vi "DropletDB-GFV.vi"(8 "error in (no error)":errorcluster, 9 "Droplets Proccesed":refnum<vi>, 10 "Data in":variant, 11 "Command In":T2=enum."Init") -> (0 "error out":errorcluster, 2 "Data out":variant)   [LabVIEW 2013]
uses:
  DbEnum.ctl
  TypeDef/MatchesAndCircles.ctl
  ConfEnum.ctl
  ConfDB.ctl
  TypeDef/Magnification.ctl
  TypeDef/GreyLevelData.ctl
  TypeDef/FreezePointData.ctl
  DropletDB.ctl
panel:
  out "Image Out 3":T1(plugin-control)
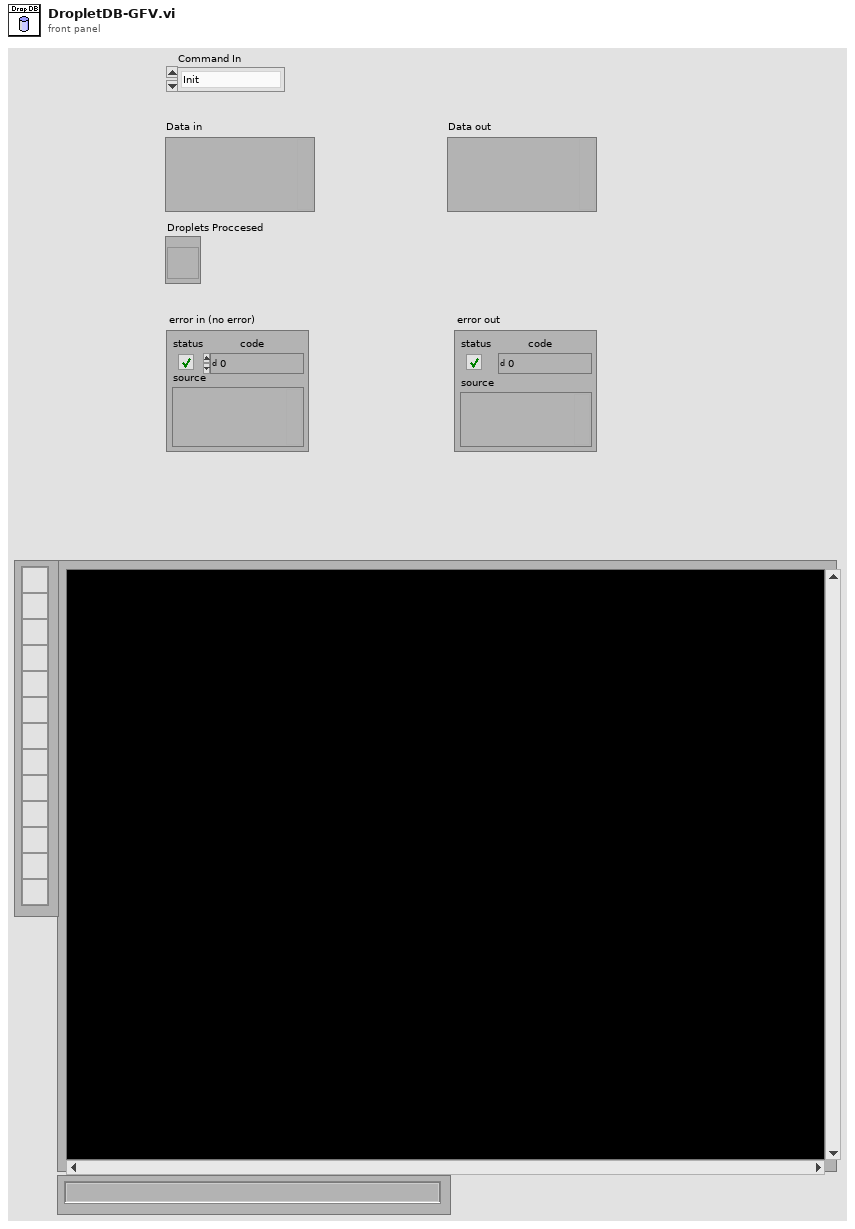
[diagram p1: front panel]
types:
  T1 = typedef "IMAQ Image.ctl" = refnum<image>
  T2 = typedef "DbEnum.ctl" = enum16{"RemoveOneDroplet", "AddOneDroplet", "Write DropletDB", "Init", "Insert Detection Result Data", "Insert Grey Level Result", "Insert Baseline Results", "AddFreezeImagesAtCertainDroplet", "UpdateIncludeDroplet", "Insert Freeze Analysis Results", "GetDropDB", "GetNoFreezedDroplets", "GetGreyLevelAndDiff", "GetGreyLevelatIndexTime", "GetDropletsBoundingBox", "GetDropletsDiameter"}
  T3 = typedef "ConfDB.ctl" = cluster{"NumberOfImages":i32, "NoImages2SaveAroundFreeze":i32, "Path":path, "NameOfPartialFile":string, "StartIndex":i32, "NumberOfStdTol":i32, "Detla t (sec)":i32, "Number of images for baseline":i32, "Temperature File Name":string, "Score":dbl, "Index number of Files":i32[], "End Index":i32, "Temperature Array":dbl[], "TStartIndex":i32, "Magnification (Microns/Pixel)":T4, "Circle Descriptor":cluster{"Min Radius":dbl, "Max Radius":dbl}}
  T4 = typedef "Magnification.ctl" = dbl
  T5 = typedef "ConfEnum.ctl" = enum16{"Init", "GetConfDB", "GetTemperatureAtIndex", "WriteConfDB", "Configure DB"}
  T6 = typedef "DropletDB.ctl" = cluster{"ImageFreezeIndex":i32, "DropIndex":i32, "Position":cluster{"x":sgl, "y":sgl}, "Bounding Box":cluster{"x":sgl, "y":sgl}[], "Score":sgl, "GreyLevelInBoundingBox":dbl[], "GLDifference":dbl[], "Baseline level":dbl, "Peak":cluster{"Value":dbl, "Index":u32}, "Peak Onset":cluster{"Value":dbl, "Index":u32}, "FreezeFileName":string, "FreezeAbsTime":timestamp, "FreezeTemperature":dbl, "ImageIndexArray":u32[], "Freeze Point Found":bool, "Baseline std":dbl, "FreezedImageArray":cluster{"Image":u8[][]}[], "Include Droplet":bool, "Remark":string, "Freeze Rel Time":u32[], "Diameter (microns)":dbl}[]
  T7 = typedef "GreyLevelData.ctl" = cluster{"Grey Level":dbl[], "Grey level diff":dbl[], "ImageIndex":u32, "Drop Index":u32}
  T8 = typedef "FreezePointData.ctl" = cluster{"Freeze YesNo":cluster{"Freeze Grey Diff value":dbl, "Freeze Point Found":bool, "Freeze Indices":u32[]}[], "Rel Time":u32[]}
  T9 = cluster{"DropletBaseline":dbl[], "DropletBaselineSTD":dbl[]}
  T10 = typedef "MatchesAndCircles.ctl" = cluster{"Matches (pixel)":cluster{"Position":cluster{"x":sgl, "y":sgl}, "Angle":sgl, "Scale":sgl, "Score":sgl, "Bounding Box":cluster{"x":sgl, "y":sgl}[]}[], "Circles (Calibrated)":cluster{"Position":cluster{"X":sgl, "Y":sgl}, "Radius":dbl, "Score":dbl}[]}
  T11 = cluster{"Position":cluster{"x":sgl, "y":sgl}, "Angle":sgl, "Scale":sgl, "Score":sgl, "Bounding Box":cluster{"x":sgl, "y":sgl}[]}[]
  T12 = cluster{"Position":cluster{"X":sgl, "Y":sgl}, "Radius":dbl, "Score":dbl}[]
  T13 = cluster{"ImageFreezeIndex":i32, "DropIndex":i32, "Position":cluster{"x":sgl, "y":sgl}, "Bounding Box":cluster{"x":sgl, "y":sgl}[], "Score":sgl, "GreyLevelInBoundingBox":dbl[], "GLDifference":dbl[], "Baseline level":dbl, "Peak":cluster{"Value":dbl, "Index":u32}, "Peak Onset":cluster{"Value":dbl, "Index":u32}, "FreezeFileName":string, "FreezeAbsTime":timestamp, "FreezeTemperature":dbl, "ImageIndexArray":u32[], "Freeze Point Found":bool, "Baseline std":dbl, "FreezedImageArray":cluster{"Image":u8[][]}[], "Include Droplet":bool, "Remark":string, "Freeze Rel Time":u32[], "Diameter (microns)":dbl}
  T14 = cluster{"Global Rectangle":i32[], "Contours":cluster{"Contour Type":u32, "ROI Type":u32, "Points":i32[]}[]}
  T15 = typedef "IMAQ Circle" = cluster{"Center X":i32, "Center Y":i32, "Inner Radius":i32, "Outer Radius":i32, "Start Angle":dbl, "End Angle":dbl}
  T16 = cluster{"Freeze Grey Diff value":dbl, "Freeze Point Found":bool, "Freeze Indices":u32[]}[]
  T17 = cluster{"ImageFreezeIndex":i32, "DropIndex":i32, "Position":cluster{"x":sgl, "y":sgl}, "Bounding Box":cluster{"x":sgl, "y":sgl}[], "Score":sgl, "GreyLevelInBoundingBox":dbl[], "GLDifference":dbl[], "Baseline level":dbl, "Peak":cluster{"Value":dbl, "Index":u32}, "Peak Onset":cluster{"Value":dbl, "Index":u32}, "FreezeFileName":string, "FreezeAbsTime":timestamp, "FreezeTemperature":dbl, "ImageIndexArray":u32[], "Freeze Point Found":bool, "Baseline std":dbl, "FreezedImageArray":cluster{"Image":u8[][]}[], "Include Droplet":bool, "Remark":string, "Freeze Rel Time":u32[], "Diameter (microns)":dbl}[]
  T18 = cluster{"ImageIndexArray":u32[], "GreyLevelInBoundingBox":dbl[][], "GLDifference":dbl[][]}
  T19 = typedef "Image Type" = u32
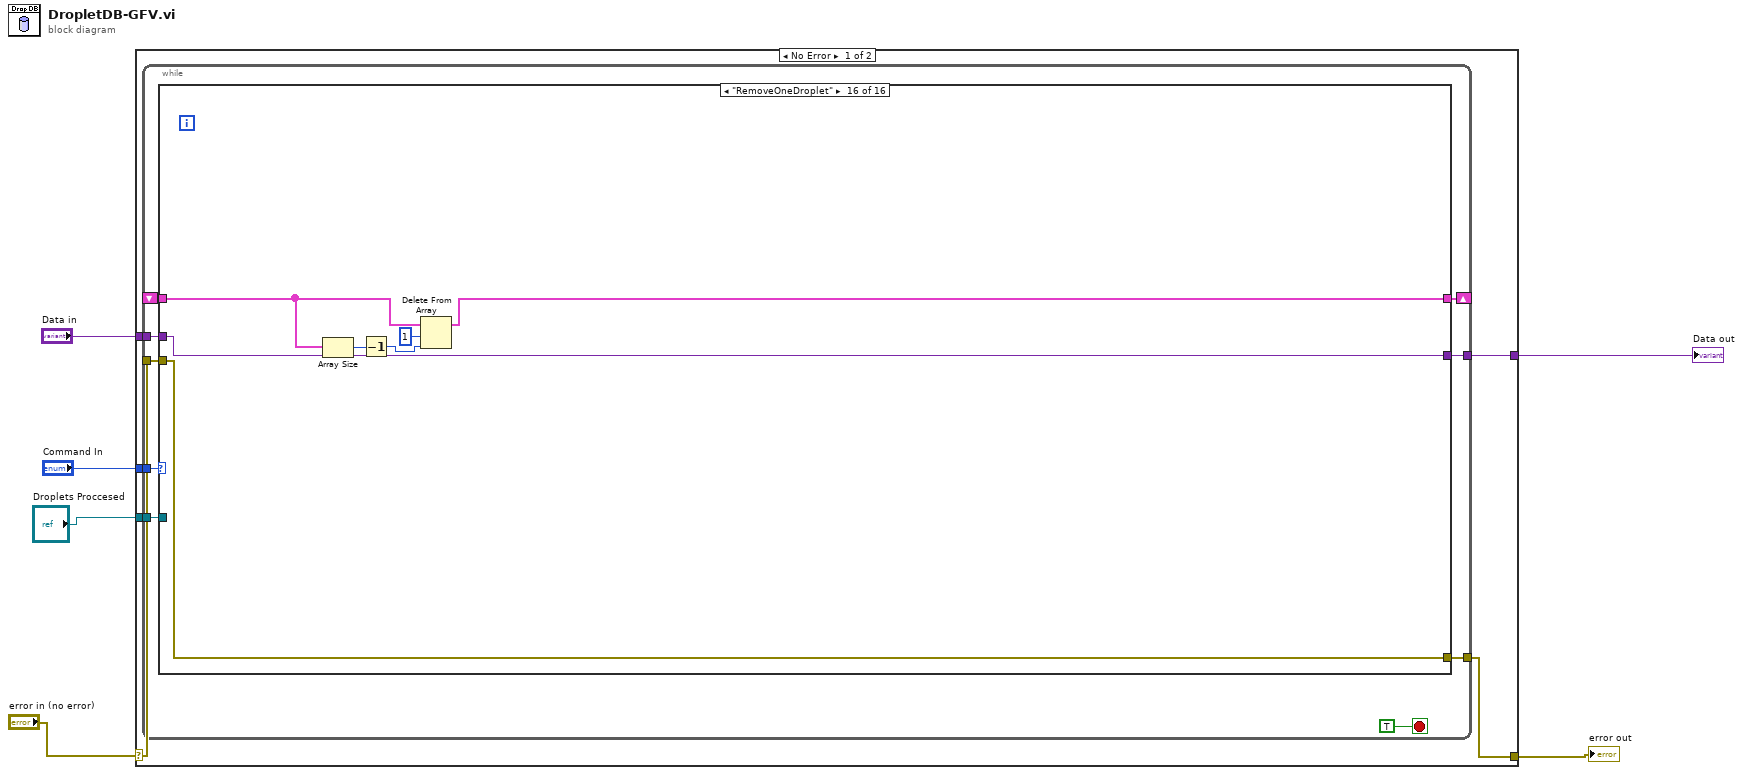
[diagram p0: block diagram]
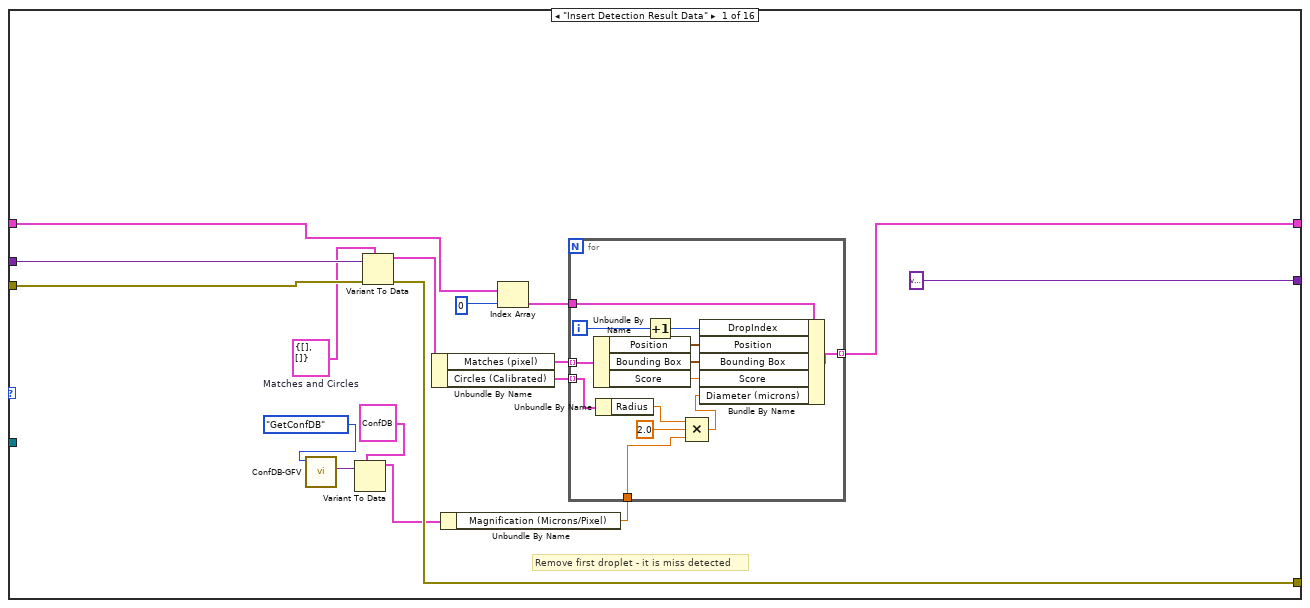
[diagram p2: hidden frame]
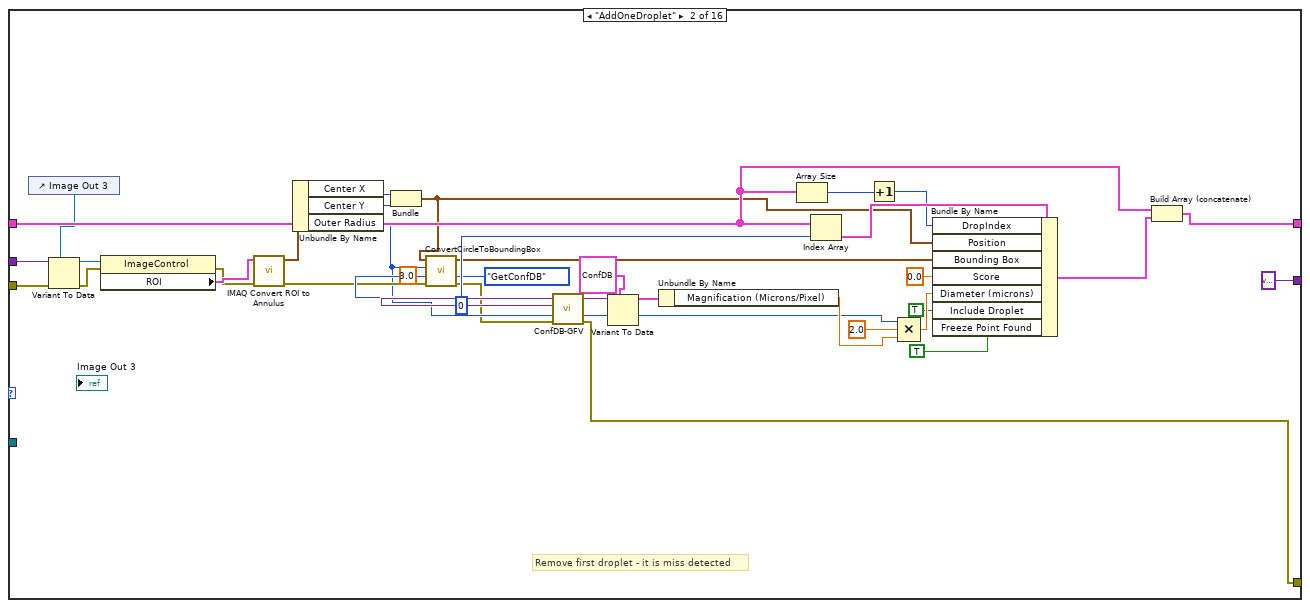
[diagram p3: hidden frame]
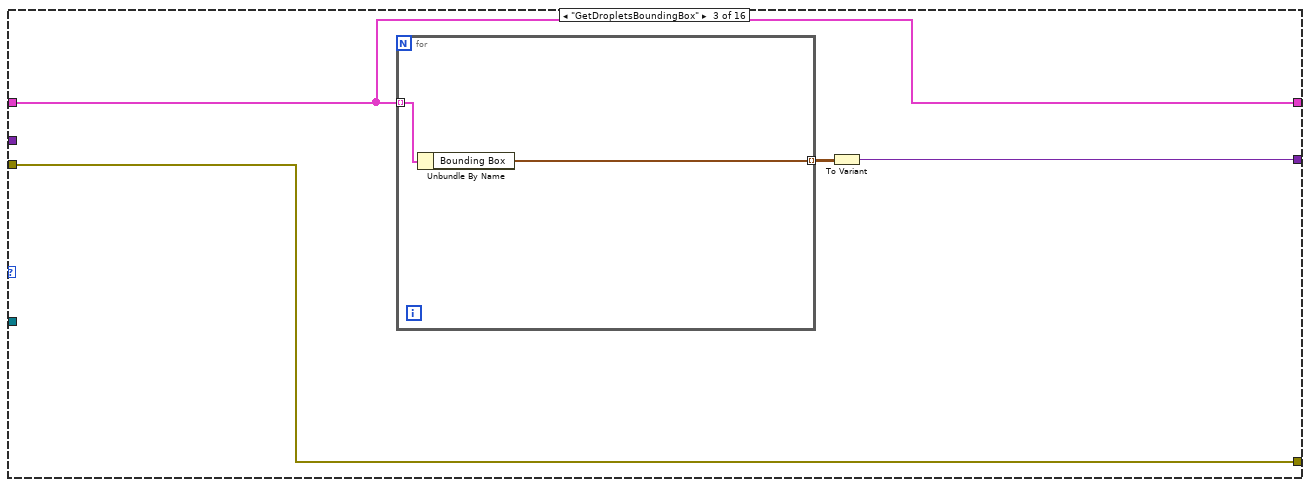
[diagram p4: hidden frame]
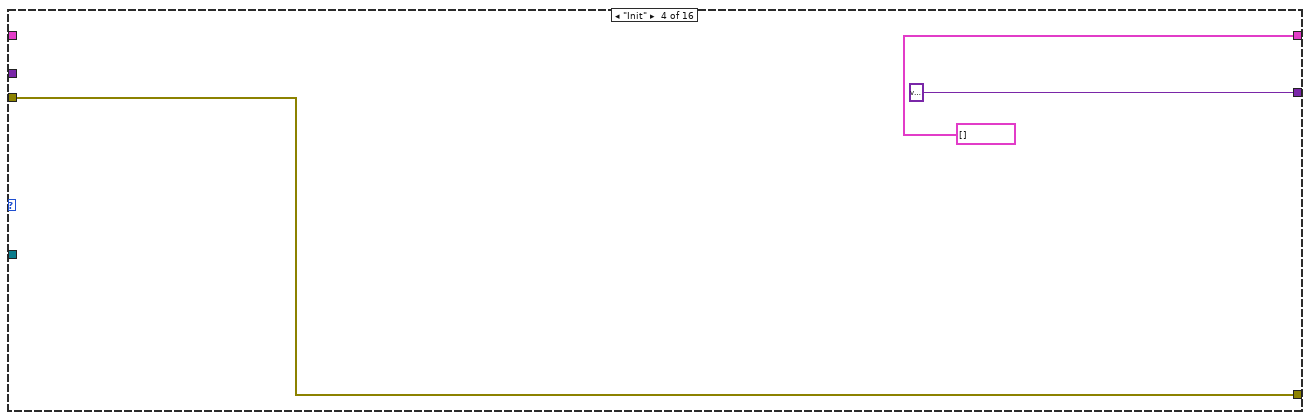
[diagram p5: hidden frame]
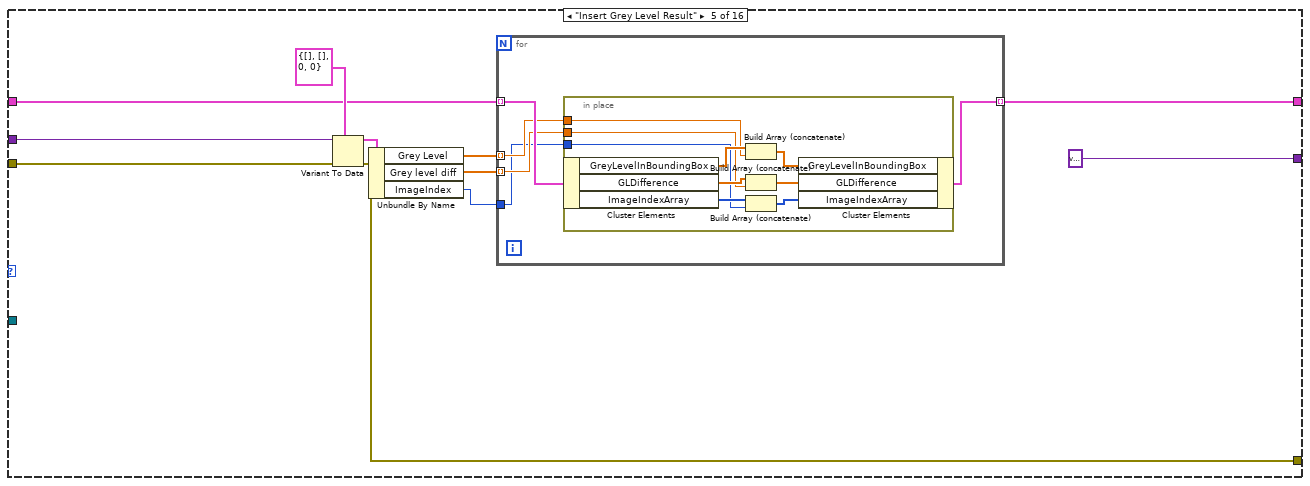
[diagram p6: hidden frame]
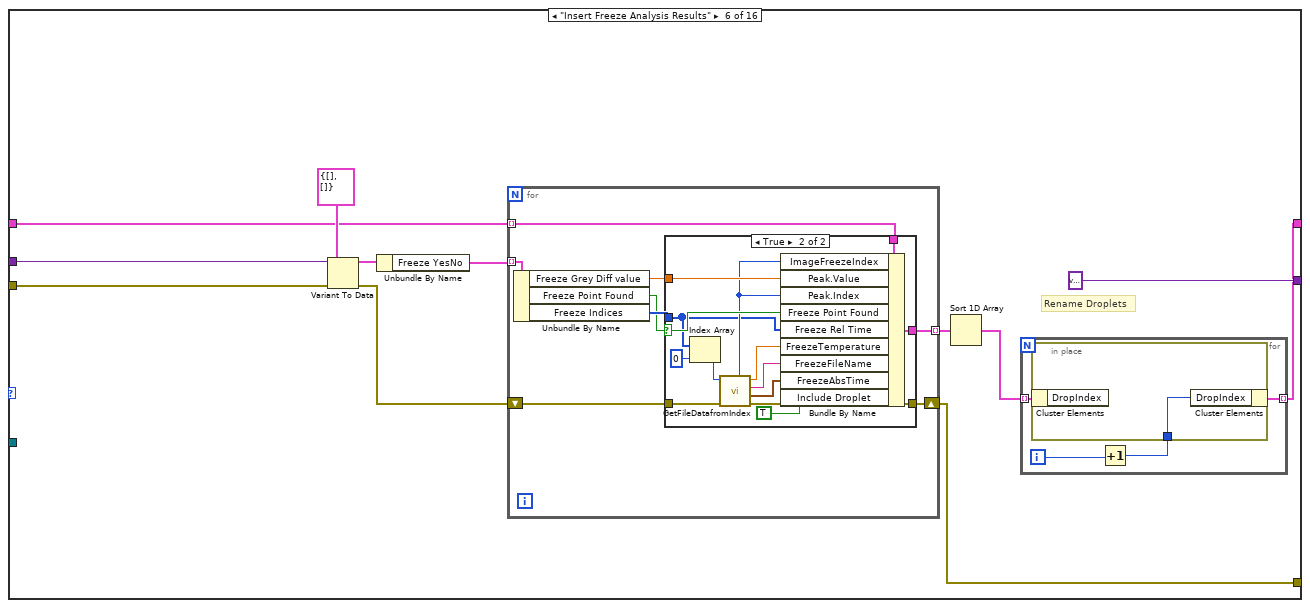
[diagram p7: hidden frame]
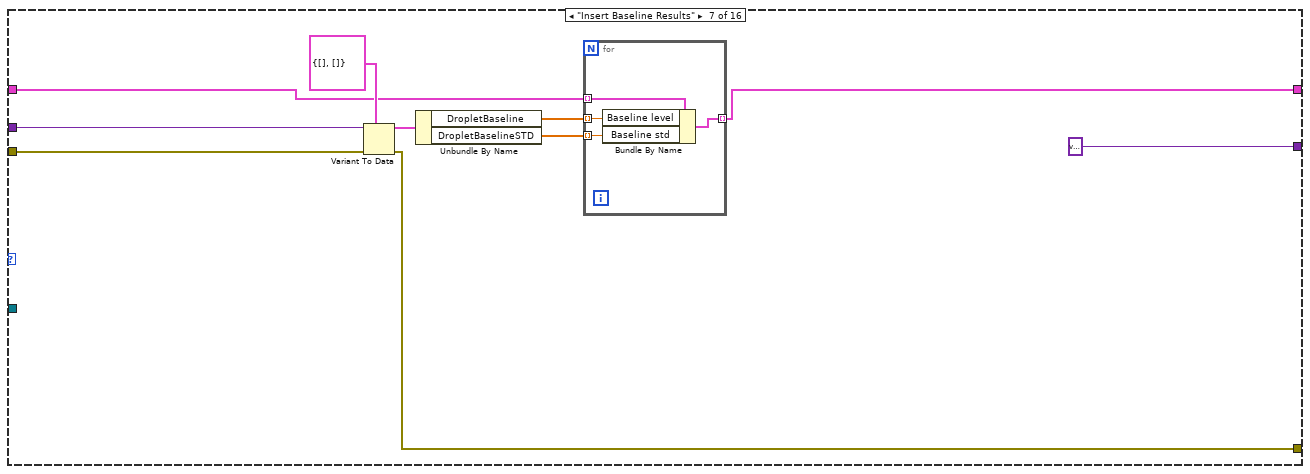
[diagram p9: hidden frame]
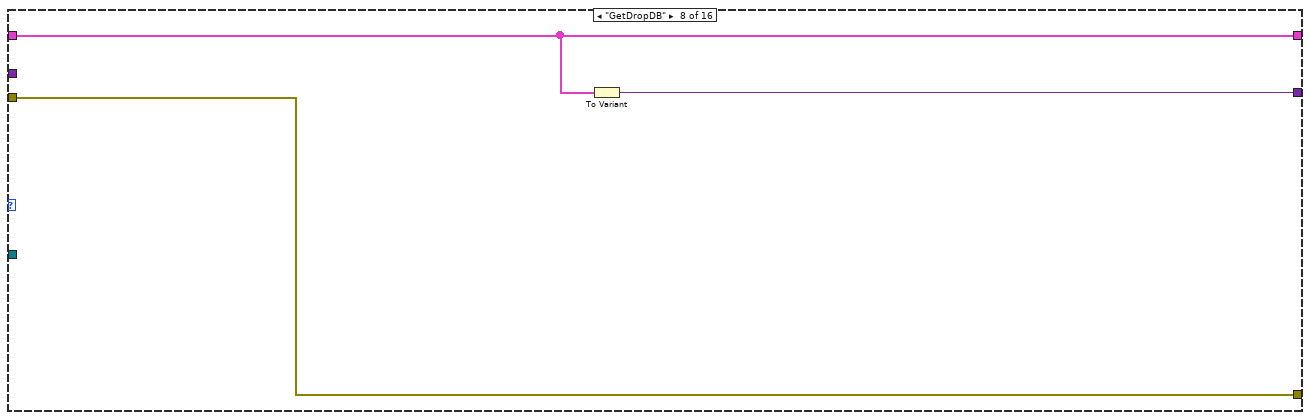
[diagram p10: hidden frame]
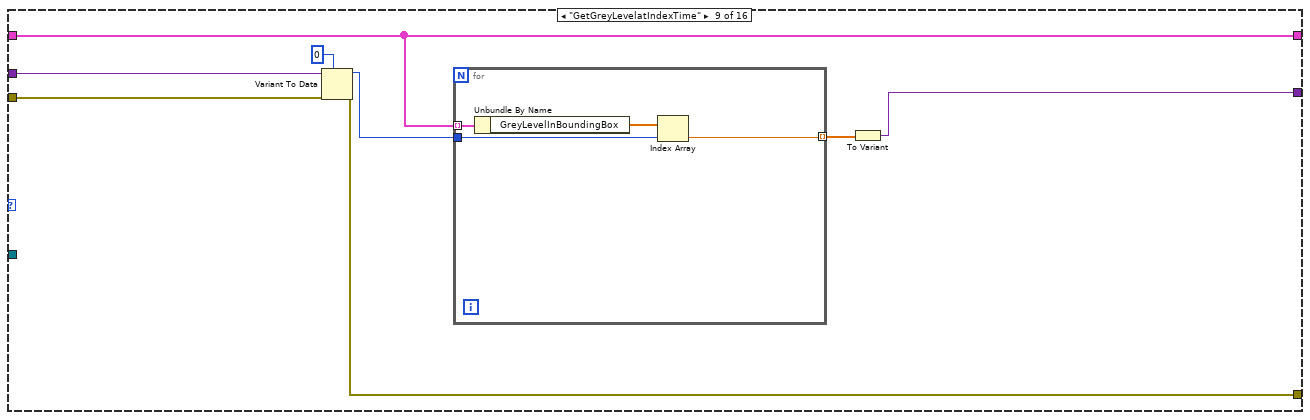
[diagram p11: hidden frame]
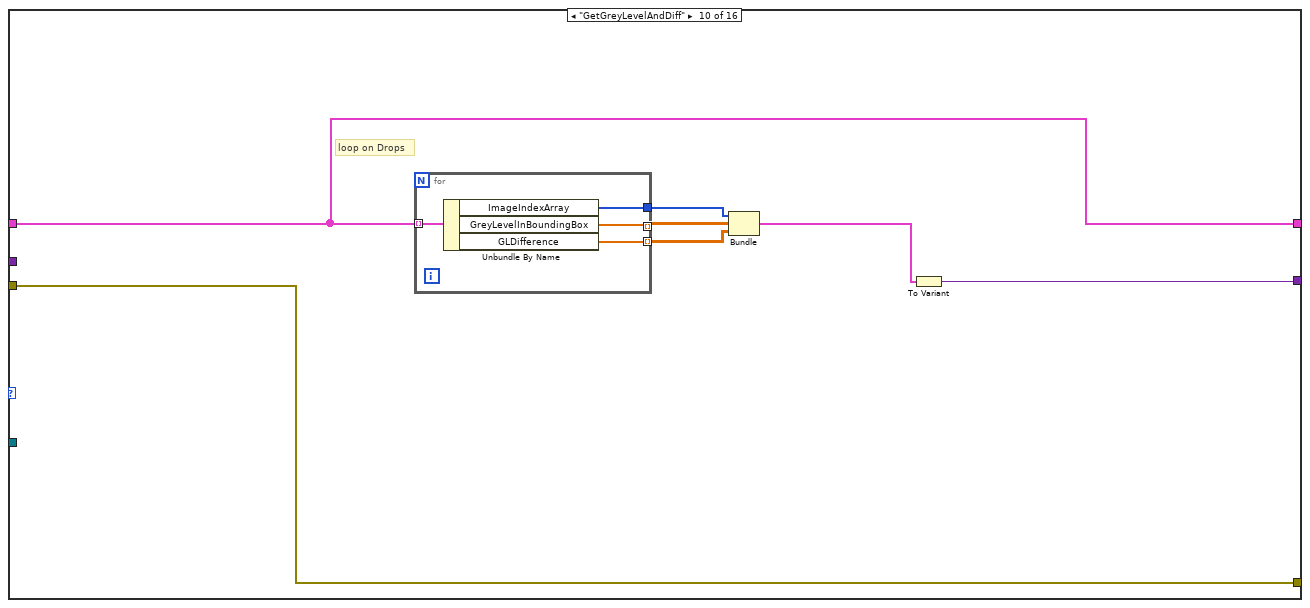
[diagram p12: hidden frame]
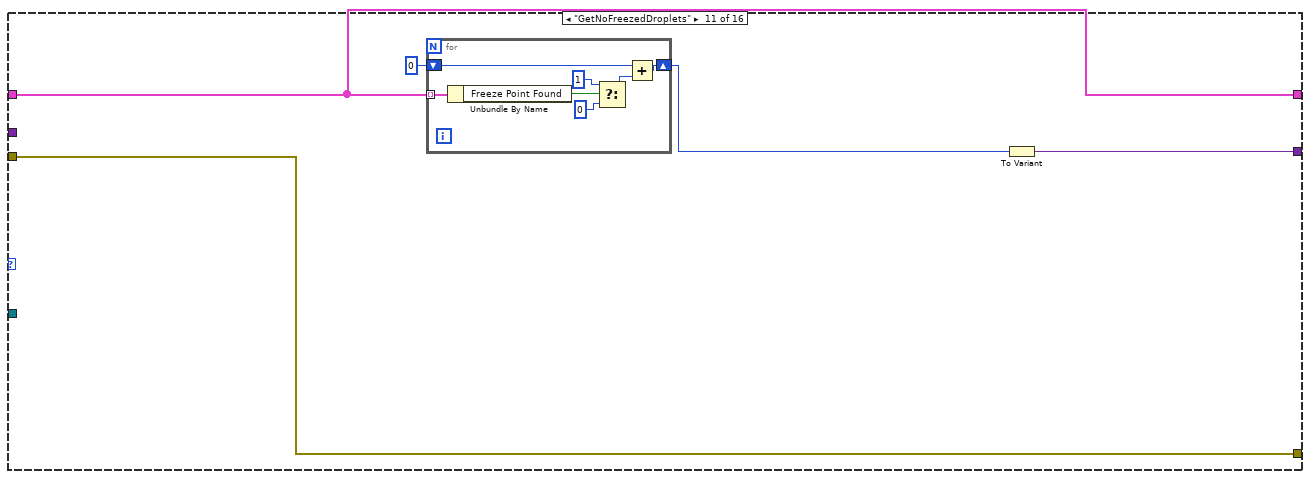
[diagram p13: hidden frame]
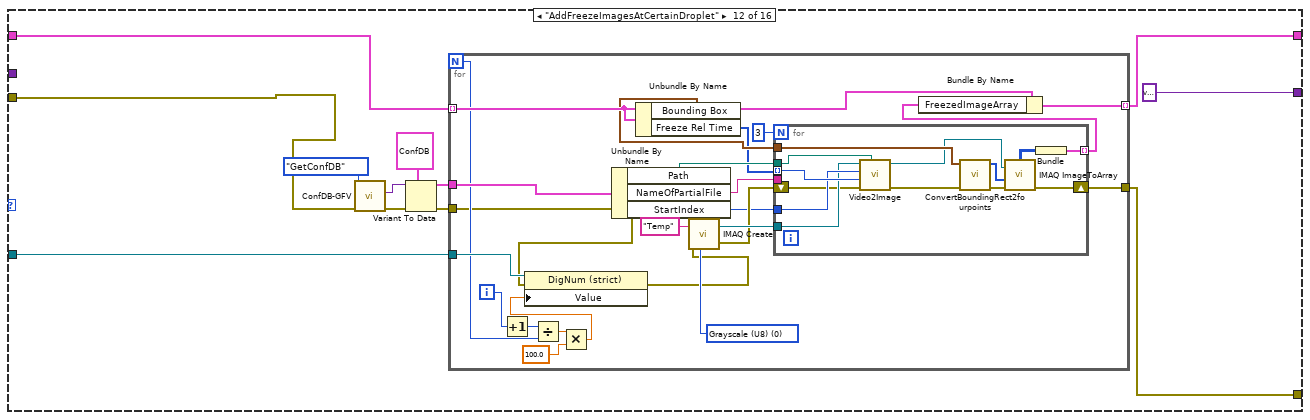
[diagram p14: hidden frame]
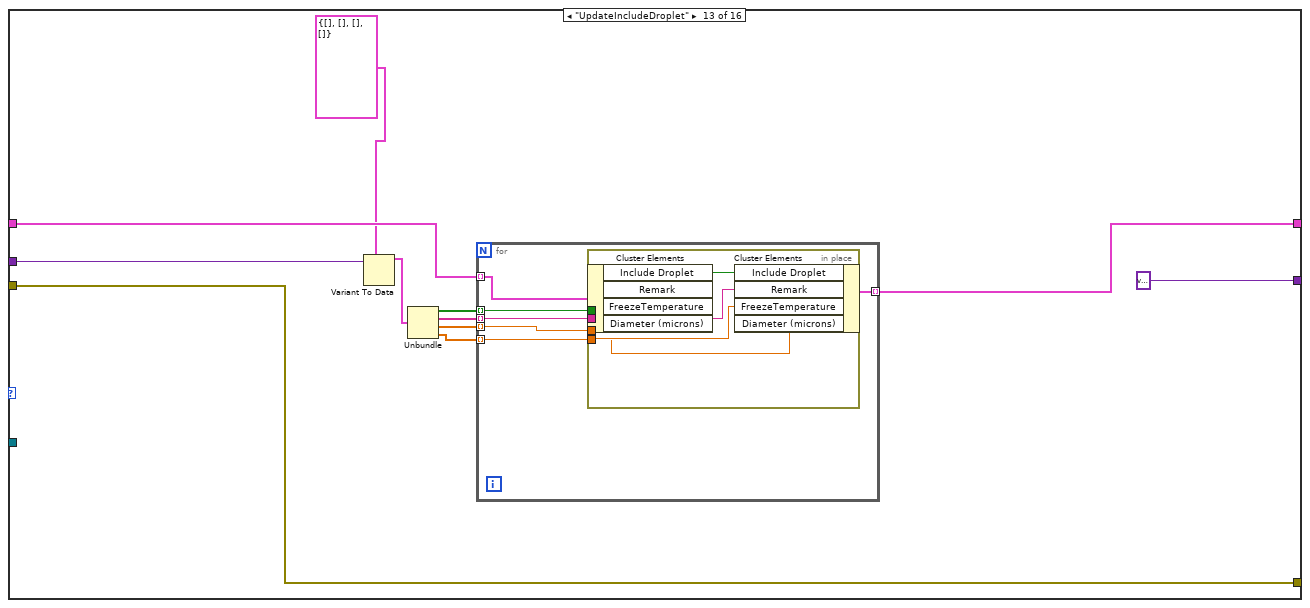
[diagram p15: hidden frame]
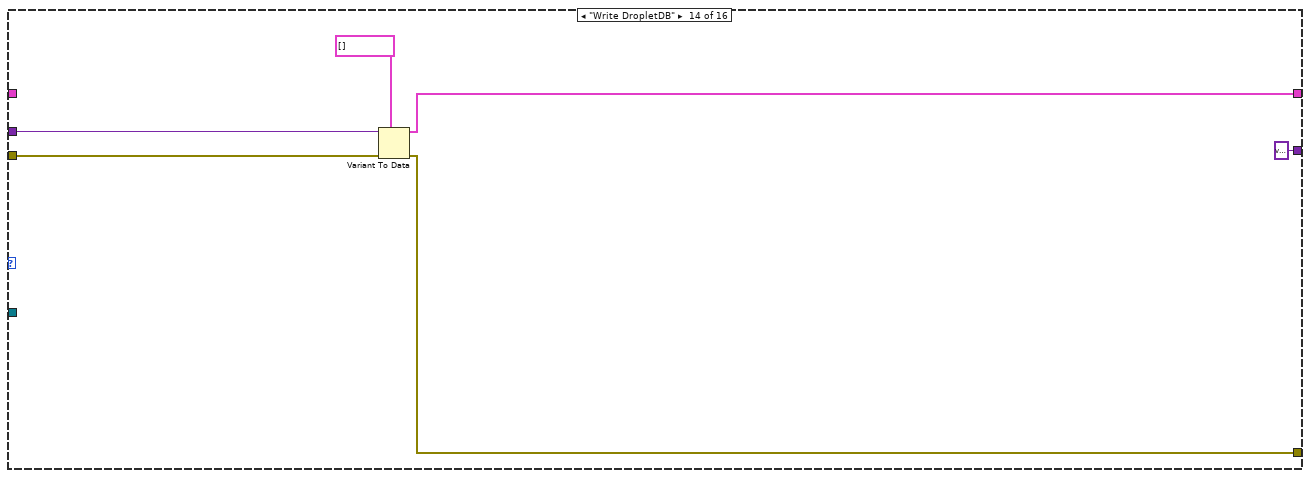
[diagram p16: hidden frame]
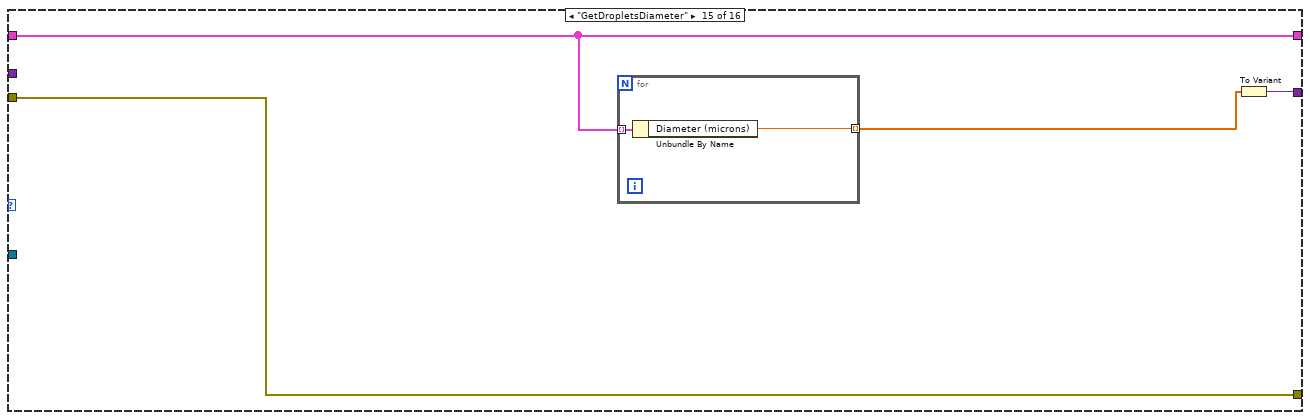
[diagram p17: hidden frame]
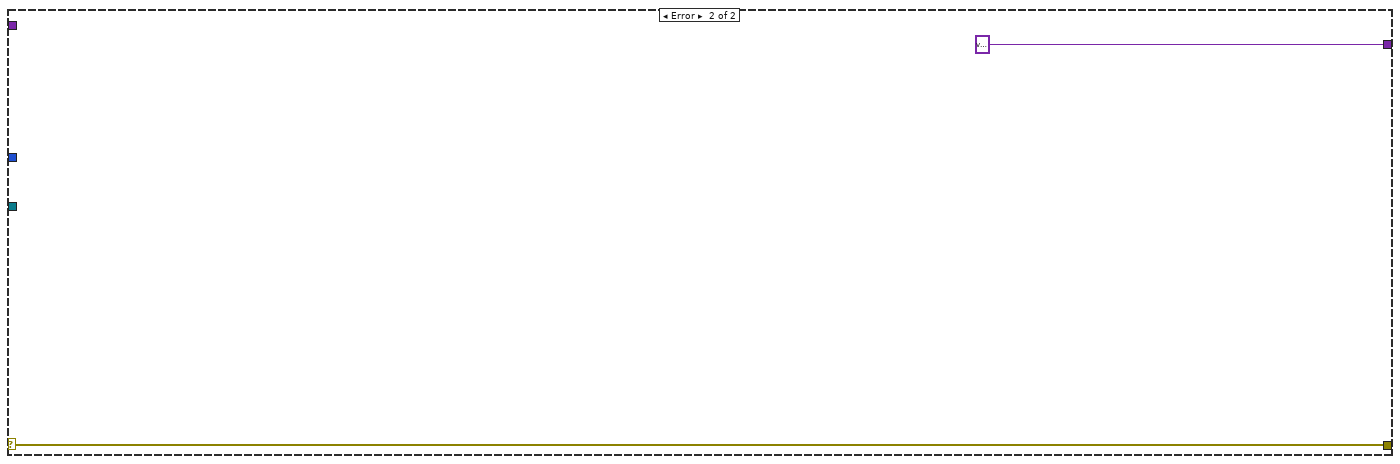
[diagram p18: hidden frame]
diagram:
  n1 = case shown="No Error" "error in (no error)" {
    selector: "error in (no error)" -> [w9 w304]
    tunnel: [w8 w304] -> w5
    tunnel: "Command In" -> [w12 _]
    tunnel: "Data in" -> [w11 _]
    tunnel: [w10 variant ("Variant")] -> w2
    tunnel: "Droplets Proccesed" -> [w7 _]
    frame No Error {
      n2 = while {
        tunnel: w12 -> [w20]
        shift-right: [w19] -> _
        shift-left: _ -> [w17]
        tunnel: w11 -> [w18]
        tunnel: [w16] -> w10
        tunnel: w9 -> [w15]
        tunnel: [w14] -> w8
        tunnel: w7 -> [w13]
        stop <- TRUE stop-if-true
        n3 = case shown="\"RemoveOneDroplet\"" w20 {
          tunnel: [w34 w73 w90 T6 [] ("DropletArray") w97 w122 w164 w178 w184 w197 w205 w217 w269 w286 w292 w296] -> w19
          tunnel: w18 -> [w38 w70 _ _ w106 w132 w170 _ w186 _ _ _ w271 w289 _ w302]
          tunnel: w17 -> [w35 w77 w90 _ w100 w128 w168 w178 w184 w197 w205 w216 w270 _ w292 w299]
          tunnel: [variant ("Variant") variant ("Variant") w88 variant ("Variant") variant ("Variant") variant ("Variant") variant ("Variant") w177 w181 w196 w204 variant ("Variant") variant ("Variant") variant ("Variant") w291 w302] -> w16
          tunnel: w15 -> [w32 w66 w87 w93 w102 w131 w171 w176 w180 w191 w202 w215 w273 w288 w293 w301]
          tunnel: [w31 w72 w87 w93 w101 w125 w162 w176 w179 w191 w202 w218 w273 w285 w293 w301] -> w14
          tunnel: w13 -> [_ _ _ _ _ _ _ _ _ _ _ w214 _ _ _ _]
          frame "Insert Detection Result Data" {
            w30 = T10 {"Matches (pixel)"=[], "Circles (Calibrated)"=[]}  # Matches and Circles
            # "Remove first droplet - it is miss detected"
            n4 = call "ConfDB-GFV.vi"("Command In"=ConfEnum."GetConfDB") -> ("Data out"=w26:variant)  [unwired: 9 in, 1 out]
            n5 = Variant To Data(type=T3 {"NumberOfImages"=0, "NoImages2SaveAroundFreeze"=0, "Path"=path "", "NameOfPartialFile"="", "StartIndex"=0, "NumberOfStdTol"=0, "Detla t (sec)"=0, "Number of images for baseline"=0, "Temperature File Name"="", "Score"=0.0, "Index number of Files"=[], "End Index"=0, "Temperature Array"=[], "TStartIndex"=0, "Magnification (Microns/Pixel)"=0.0, "Circle Descriptor"={"Min Radius"=0.0, "Max Radius"=0.0}} ("ConfDB"), Variant=w26) -> (data=w23:T3)  [unwired: 1 in, 1 out]
            n6 = Variant To Data(error in=w32, type=w30, Variant=w38) -> (data=w29:T10, error out=w31:errorcluster)
            n7 = Unbundle By Name(w29) -> ("Matches (pixel)"=w28:T11, "Circles (Calibrated)"=w27:T12)
            n8 = Unbundle By Name(w23) -> ("Magnification (Microns/Pixel)"=w22:T4)
            n9 = Index Array(array=w35, index=0) -> (element=w36:T13)
            n10 = for {
              tunnel: w28 -> [w46] mode=indexing
              tunnel: [w48] -> w34 mode=indexing
              tunnel: w36 -> [w47]
              tunnel: w27 -> [w43] mode=indexing
              tunnel: w22 -> [w40]
              i -> [w45]
              n11 = Unbundle By Name(w46) -> ("Position"=w51:cluster{"x":sgl, "y":sgl}, "Bounding Box"=w50:cluster{"x":sgl, "y":sgl}[], "Score"=w49:sgl)
              n12 = Unbundle By Name(w43) -> ("Radius"=w42:dbl)
              n13 = Increment(x=w45) -> (x+1=w44:i32)
              n14 = Compound Arithmetic op=MULTIPLY(w42, 2.0 ("value"), w40) -> (w39:T4)
              n15 = Bundle By Name(cluster=w47, "DropIndex"=w44, "Position"=w51, "Bounding Box"=w50, "Score"=w49, "Diameter (microns)"=w39) -> (w48:T13)
            }
          }
          frame "AddOneDroplet" {
            # "Remove first droplet - it is miss detected"
            n16 = control-ref of="Image Out 3"() -> (w67:refnum<vi>)
            n17 = Variant To Data(error in=w66, type=w67, Variant=w70) -> (data=w69:refnum<vi>, error out=w65:errorcluster)
            n18 = property on="Property Node" class="ImageControl"(reference=w69, error in=w65) -> (error out=w64:errorcluster, "ROI"=w68:T14)  [unwired: 1 out]
            n19 = call "IMAQ Convert ROI to Annulus"("error in (no error)"=w64, "ROI Descriptor"=w68) -> ("error out"=w60:errorcluster, "Annulus"=w63:T15)  [unwired: 7 in]
            n20 = Unbundle By Name(w63) -> ("Center X"=w62:i32, "Center Y"=w61:i32, "Outer Radius"=w56:i32)
            n21 = Bundle("Center X"=w62, "Center Y"=w61) -> (w59:cluster{"Center X":i32, "Center Y":i32})  [unwired: 1 in]
            n22 = call "ConvertCircleToBoundingBox.vi"("error in (no error)"=w60, "InflateBoxbyPixelNo"=3.0, "Radius"=w56, "Position"=w59) -> ("error out"=w54:errorcluster, "Bounding Box"=w57:cluster{"x":sgl, "y":sgl}[])  [unwired: 6 in]
            n23 = call "ConfDB-GFV.vi"("error in (no error)"=w54, "Command In"=ConfEnum."GetConfDB") -> ("error out"=w72:errorcluster, "Data out"=w84:variant)  [unwired: 8 in]
            n24 = Variant To Data(type=T3 {"NumberOfImages"=0, "NoImages2SaveAroundFreeze"=0, "Path"=path "", "NameOfPartialFile"="", "StartIndex"=0, "NumberOfStdTol"=0, "Detla t (sec)"=0, "Number of images for baseline"=0, "Temperature File Name"="", "Score"=0.0, "Index number of Files"=[], "End Index"=0, "Temperature Array"=[], "TStartIndex"=0, "Magnification (Microns/Pixel)"=0.0, "Circle Descriptor"={"Min Radius"=0.0, "Max Radius"=0.0}} ("ConfDB"), Variant=w84) -> (data=w81:T3)  [unwired: 1 in, 1 out]
            n25 = Unbundle By Name(w81) -> ("Magnification (Microns/Pixel)"=w80:T4)
            n26 = Array Size(array=w77) -> (size(s)=w75:i32)
            n27 = Index Array(array=w77, index=0) -> (element=w79:T13)
            n28 = Increment(x=w75) -> (x+1=w76:i32)
            n29 = Compound Arithmetic op=MULTIPLY(w56, 2.0 ("value"), w80) -> (w55:T4)
            n30 = Bundle By Name(cluster=w79, "DropIndex"=w76, "Position"=w59, "Bounding Box"=w57, "Score"=sgl 0.0, "Diameter (microns)"=w55, "Include Droplet"=TRUE, "Freeze Point Found"=TRUE) -> (w74:T13)
            n31 = Build Array (concatenate)(w77, w74) -> (w73:T6)
          }
          frame "GetDropletsBoundingBox" {
            n32 = for {
              tunnel: w90 -> [w92] mode=indexing
              tunnel: [w91] -> w89 mode=indexing
              n33 = Unbundle By Name(w92) -> ("Bounding Box"=w91:cluster{"x":sgl, "y":sgl}[])
            }
            n34 = To Variant(anything=w89) -> (Variant=w88:variant)
          }
          frame "Init" {
          }
          frame "Insert Grey Level Result" {
            n35 = Variant To Data(error in=w102, type=T7 {"Grey Level"=[], "Grey level diff"=[], "ImageIndex"=0, "Drop Index"=0} ("Cluster"), Variant=w106) -> (data=w104:T7, error out=w101:errorcluster)
            n36 = Unbundle By Name(w104) -> ("Grey Level"=w99:dbl[], "Grey level diff"=w98:dbl[], "ImageIndex"=w96:u32)
            n37 = for {
              tunnel: w100 -> [w111] mode=indexing
              tunnel: w99 -> [w110] mode=indexing
              tunnel: w98 -> [w109] mode=indexing
              tunnel: [w108] -> w97 mode=indexing
              tunnel: w96 -> [w107]
              n38 = in-place {
                in-place-border: w110 -> [w118]
                in-place-border: w109 -> [w115]
                in-place-border: w107 -> [w112]
                n39 = in-place-cluster #1(w111) -> ("GreyLevelInBoundingBox"=w120:dbl[], "GLDifference"=w117:dbl[], "ImageIndexArray"=w114:u32[])
                n40 = Build Array (concatenate)(w120, w118) -> (w119:dbl[])
                n41 = Build Array (concatenate)(w117, w115) -> (w116:dbl[])
                n42 = Build Array (concatenate)(w114, w112) -> (w113:u32[])
                n43 = in-place-cluster #1("GreyLevelInBoundingBox"=w119, "GLDifference"=w116, "ImageIndexArray"=w113) -> (w108:T13)
              }
            }
          }
          frame "Insert Freeze Analysis Results" {
            # "Rename Droplets"
            n44 = Variant To Data(error in=w131, type=T8 {"Freeze YesNo"=[], "Rel Time"=[]} ("Freeze YesNo"), Variant=w132) -> (data=w127:T8, error out=w121:errorcluster)
            n45 = Unbundle By Name(w127) -> ("Freeze YesNo"=w126:T16)
            n46 = for {
              tunnel: w126 -> [w145] mode=indexing
              tunnel: w128 -> [w144] mode=indexing
              tunnel: [w142] -> w124 mode=indexing
              shift-right: [w140] -> w125
              shift-left: w121 -> [w141]
              n47 = Unbundle By Name(w145) -> ("Freeze Grey Diff value"=w143:dbl, "Freeze Point Found"=w138:bool, "Freeze Indices"=w139:u32[])
              n48 = case shown="True" w138 {
                selector: w138 -> [_ w153]
                tunnel: w144 -> [w147 w161]
                tunnel: w143 -> [_ w160]
                tunnel: [w147 w159] -> w142
                tunnel: w141 -> [w146 w158]
                tunnel: [w146 w157] -> w140
                tunnel: w139 -> [_ w150]
                frame False {
                }
                frame True {
                  n49 = Index Array(array=w150, index=0) -> (element=w148:u32)
                  n50 = call "GetFileDatafromIndex.vi"("Error In"=w158, "DuplicateFilteredIndex"=w148) -> ("Error Out"=w157:errorcluster, "FreezeAbsTime"=w154:timestamp, "FreezeFileName"=w155:string, "FreezeTemperature"=w156:dbl, "Peak index"=w152:u32)  [unwired: 5 in]
                  n51 = Bundle By Name(cluster=w161, "ImageFreezeIndex"=w152, "Peak.Value"=w160, "Peak.Index"=w152, "Freeze Point Found"=w153, "Freeze Rel Time"=w150, "FreezeTemperature"=w156, "FreezeFileName"=w155, "FreezeAbsTime"=w154, "Include Droplet"=TRUE) -> (w159:T13)
                }
              }
            }
            n52 = Sort 1D Array(array=w124) -> (sorted array=w123:T17)
            n53 = for {
              tunnel: w123 -> [w136] mode=indexing
              tunnel: [w135] -> w122 mode=indexing
              i -> [w134]
              n54 = Increment(x=w134) -> (x+1=w133:i32)
              n55 = in-place {
                in-place-border: w133 -> [w137]
                n56 = in-place-cluster #2(w136) -> ()  [unwired: 1 out]
                n57 = in-place-cluster #2("DropIndex"=w137) -> (w135:T13)
              }
            }
          }
          frame "Insert Baseline Results" {
            n58 = Variant To Data(error in=w171, type=T9 {"DropletBaseline"=[], "DropletBaselineSTD"=[]} ("output cluster"), Variant=w170) -> (data=w167:T9, error out=w162:errorcluster)
            n59 = Unbundle By Name(w167) -> ("DropletBaseline"=w166:dbl[], "DropletBaselineSTD"=w165:dbl[])
            n60 = for {
              tunnel: w168 -> [w175] mode=indexing
              tunnel: w166 -> [w174] mode=indexing
              tunnel: w165 -> [w172] mode=indexing
              tunnel: [w173] -> w164 mode=indexing
              n61 = Bundle By Name(cluster=w175, "Baseline level"=w174, "Baseline std"=w172) -> (w173:T13)
            }
          }
          frame "GetDropDB" {
            n62 = To Variant(anything=w178) -> (Variant=w177:variant)
          }
          frame "GetGreyLevelatIndexTime" {
            n63 = Variant To Data(error in=w180, type=0 ("x-y"), Variant=w186) -> (data=w183:i32, error out=w179:errorcluster)
            n64 = for {
              tunnel: w184 -> [w190] mode=indexing
              tunnel: w183 -> [w188]
              tunnel: [w187] -> w182 mode=indexing
              n65 = Unbundle By Name(w190) -> ("GreyLevelInBoundingBox"=w189:dbl[])
              n66 = Index Array(array=w189, index=w188) -> (element=w187:dbl)
            }
            n67 = To Variant(anything=w182) -> (Variant=w181:variant)
          }
          frame "GetGreyLevelAndDiff" {
            # "loop on Drops"
            n68 = for {
              tunnel: w197 -> [w201] mode=indexing
              tunnel: [w200] -> w194 mode=indexing
              tunnel: [w199] -> w193 mode=indexing
              tunnel: [w198] -> w195
              n69 = Unbundle By Name(w201) -> ("ImageIndexArray"=w198:u32[], "GreyLevelInBoundingBox"=w200:dbl[], "GLDifference"=w199:dbl[])
            }
            n70 = Bundle("ImageIndexArray"=w195, "GreyLevelInBoundingBox"=w194, "GLDifference"=w193) -> (w192:T18)  [unwired: 1 in]
            n71 = To Variant(anything=w192) -> (Variant=w196:variant)
          }
          frame "GetNoFreezedDroplets" {
            n72 = for {
              tunnel: w205 -> [w213] mode=indexing
              shift-right: [w208] -> w203
              shift-left: u32 0 -> [w207]
              n73 = Unbundle By Name(w213) -> ("Freeze Point Found"=w212:bool)
              n74 = Select(t=u32 1, s=w212, f=u32 0) -> (s? t:f=w211:u32)
              n75 = Add(x=w207, y=w211) -> (x+y=w208:u32)
            }
            n76 = To Variant(anything=w203) -> (Variant=w204:variant)
          }
          frame "AddFreezeImagesAtCertainDroplet" {
            n77 = call "ConfDB-GFV.vi"("error in (no error)"=w215, "Command In"=ConfEnum."GetConfDB") -> ("error out"=w222:errorcluster, "Data out"=w223:variant)  [unwired: 8 in]
            n78 = Variant To Data(error in=w222, type=T3 {"NumberOfImages"=0, "NoImages2SaveAroundFreeze"=0, "Path"=path "", "NameOfPartialFile"="", "StartIndex"=0, "NumberOfStdTol"=0, "Detla t (sec)"=0, "Number of images for baseline"=0, "Temperature File Name"="", "Score"=0.0, "Index number of Files"=[], "End Index"=0, "Temperature Array"=[], "TStartIndex"=0, "Magnification (Microns/Pixel)"=0.0, "Circle Descriptor"={"Min Radius"=0.0, "Max Radius"=0.0}} ("ConfDB"), Variant=w223) -> (data=w220:T3, error out=w219:errorcluster)
            n79 = for {
              N -> [w233]
              tunnel: w220 -> [w249]
              tunnel: w219 -> [w229]
              tunnel: [w248] -> w218
              tunnel: w216 -> [w246] mode=indexing
              tunnel: [w247] -> w217 mode=indexing
              tunnel: w214 -> [w234]
              i -> [w226]
              w243 = T19 0 items=["Grayscale (U8)", "Grayscale (I16)", "Grayscale (SGL)", "Complex (CSG)", "RGB (U32)", "HSL (U32)", "RGB (U64)", "Grayscale (U16)"] ("Image Type")
              n80 = Increment(x=w226) -> (x+1=w227:i32)
              n81 = Divide(x=w227, y=w233) -> (x/y=w232:dbl)
              n82 = Multiply(x=w232, y=100.0) -> (x*y=w230:dbl)
              n83 = property class="DigNum (strict)"(reference=w234, error in=w229, "Value"=w230) -> (error out=w228:errorcluster)  [unwired: 1 out]
              n84 = Unbundle By Name(w249) -> ("Path"=w245:path, "NameOfPartialFile"=w244:string, "StartIndex"=w235:i32)
              n85 = Unbundle By Name(w246) -> ("Bounding Box"=w237:cluster{"x":sgl, "y":sgl}[], "Freeze Rel Time"=w236:u32[])
              n86 = call "IMAQ Create"("Image Name"="Temp", "Image Type"=w243, "error in (no error)"=w228) -> ("New Image"=w241:T1, "error out"=w240:errorcluster)  [unwired: 1 in, 1 out]
              n87 = for {
                N: 3 -> [_]
                tunnel: w245 -> [w252]
                tunnel: w244 -> [_]
                tunnel: w241 -> [w254]
                tunnel: [w259] -> w238 mode=indexing
                shift-right: [w258] -> w248
                shift-left: w240 -> [w253]
                tunnel: w237 -> [w257]
                tunnel: w236 -> [w256] mode=indexing
                tunnel: w235 -> [w255]
                n88 = call "Video2Image.vi"("AVI File Path"=w252, "error in (no error)"=w253, "Running Index"=w256, "Start Index"=w255, "Image In"=w254) -> ("error out"=w250:errorcluster, "Image Out"=w251:T1)  [unwired: 5 in]
                n89 = call "ConvertBoundingRect2fourpoints.vi"("Error In"=w250, "Bounding Box"=w257) -> ("Error Out"=w262:errorcluster, "Array"=w261:i32[])  [unwired: 8 in]
                n90 = call "IMAQ ImageToArray"("error in (no error)"=w262, "Optional Rectangle"=w261, "Image"=w251) -> ("error out"=w258:errorcluster, "Image Pixels (U8)"=w260:u8[][])  [unwired: 1 in, 3 out]
                n91 = Bundle("Image Pixels (U8)"=w260) -> (w259:cluster{"Image Pixels (U8)":u8[][]})  [unwired: 1 in]
              }
              n92 = Bundle By Name(cluster=w246, "FreezedImageArray"=w238) -> (w247:T13)
            }
          }
          frame "UpdateIncludeDroplet" {
            n93 = Variant To Data(type=cluster{bool[], string[], dbl[], dbl[]} {[], [], [], []} ("cluster"), Variant=w271) -> (data=w268:cluster{bool[], string[], dbl[], dbl[]})  [unwired: 1 in, 1 out]
            n94 = Unbundle(w268) -> (w267:bool[], w266:string[], w265:dbl[], w263:dbl[])
            n95 = for {
              tunnel: w270 -> [w279] mode=indexing
              tunnel: [w278] -> w269 mode=indexing
              tunnel: w267 -> [w277] mode=indexing
              tunnel: w266 -> [w276] mode=indexing
              tunnel: w265 -> [w275] mode=indexing
              tunnel: w263 -> [w274] mode=indexing
              n96 = in-place {
                in-place-border: w277 -> [w283]
                in-place-border: w276 -> [w282]
                in-place-border: w275 -> [w281]
                in-place-border: w274 -> [w280]
                n97 = in-place-cluster #3(w279) -> ()  [unwired: 4 out]
                n98 = in-place-cluster #3("Include Droplet"=w283, "Remark"=w282, "FreezeTemperature"=w281, "Diameter (microns)"=w280) -> (w278:T13)
              }
            }
          }
          frame "Write DropletDB" {
            n99 = Variant To Data(error in=w288, type=T6 [] ("DropletArray"), Variant=w289) -> (data=w286:T6, error out=w285:errorcluster)
          }
          frame "GetDropletsDiameter" {
            n100 = for {
              tunnel: w292 -> [w295] mode=indexing
              tunnel: [w294] -> w290 mode=indexing
              n101 = Unbundle By Name(w295) -> ("Diameter (microns)"=w294:dbl)
            }
            n102 = To Variant(anything=w290) -> (Variant=w291:variant)
          }
          frame "RemoveOneDroplet" {
            n103 = Array Size(array=w299) -> (size(s)=w298:i32)
            n104 = Decrement(x=w298) -> (x-1=w297:i32)
            n105 = Delete From Array(array=w299, length=1, index=w297) -> (array with subset deleted=w296:T6)  [unwired: 1 out]
          }
        }
      }
    }
    frame Error {
    }
  }
  "error out" <- w5
  "Data out" <- w2
